vi "Sine Wave.vi"() -> ()   [LabVIEW 2013]
uses:
  <vilib>/measure/NI_MABase.lvlib
panel:
  in  "signal type":T1(ring)
  in  "square wave duty cycle (%)":dbl=50.0 format="%0.2f"
  in  "amplitude":dbl=1.0 format="%0.2p"
  in  "frequency":dbl=10.0 format="%0.2p"
  in  "milliseconds to wait":u32
  out "Waveform Chart":waveform(dbl)(graph)
  in  "stop":bool
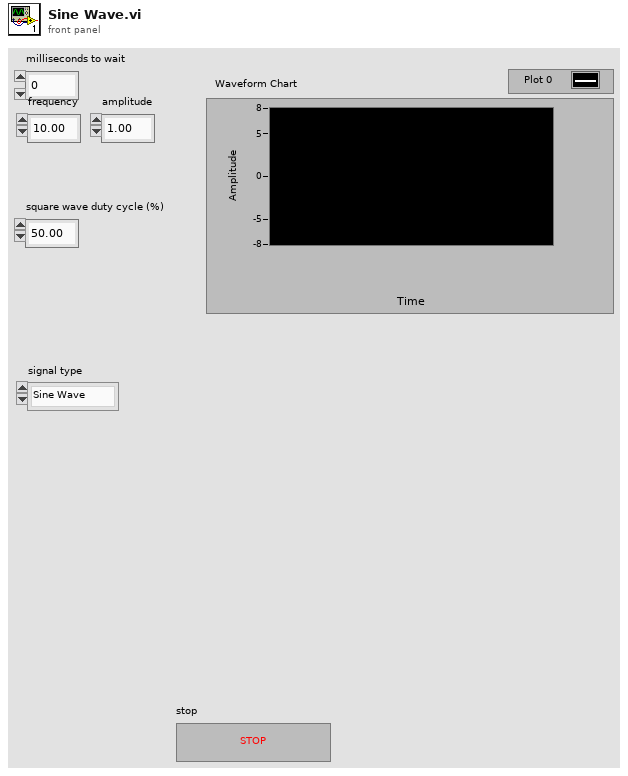
[diagram p1: front panel]
types:
  T1 = enum16{"Sine Wave", "Triangle Wave", "Square Wave", "Sawtooth Wave"}
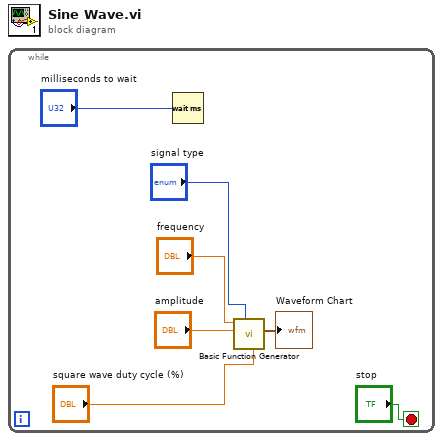
[diagram p0: block diagram]
diagram:
  n1 = while {
    stop <- "stop" stop-if-true
    n2 = Wait (ms)(milliseconds to wait="milliseconds to wait") -> ()  [unwired: 1 out]
    n3 = call <vilib>:"Basic Function Generator.vi"("square wave duty cycle (%)"="square wave duty cycle (%)", "signal type"="signal type", "amplitude"="amplitude", "frequency"="frequency") -> ("signal out"=→"Waveform Chart":waveform(dbl))  [unwired: 5 in, 2 out]
  }
